vi "DataProcessing.vi"() -> ()   [LabVIEW 2018]
panel:
  out "kat obrotu całkowity":dbl
  out "dystans przebyty x":dbl
  out "kat poł. serwomoechanizmu":dbl
  out "kat pomiaru":dbl
  out "odleglosc pomiaru":dbl
  out "dystans przebyty y":dbl
  out "XY Graph":cluster{dbl[], dbl[]}(graph)
  in  "Port":u16
  in  "Address":string
  in  "stop":bool
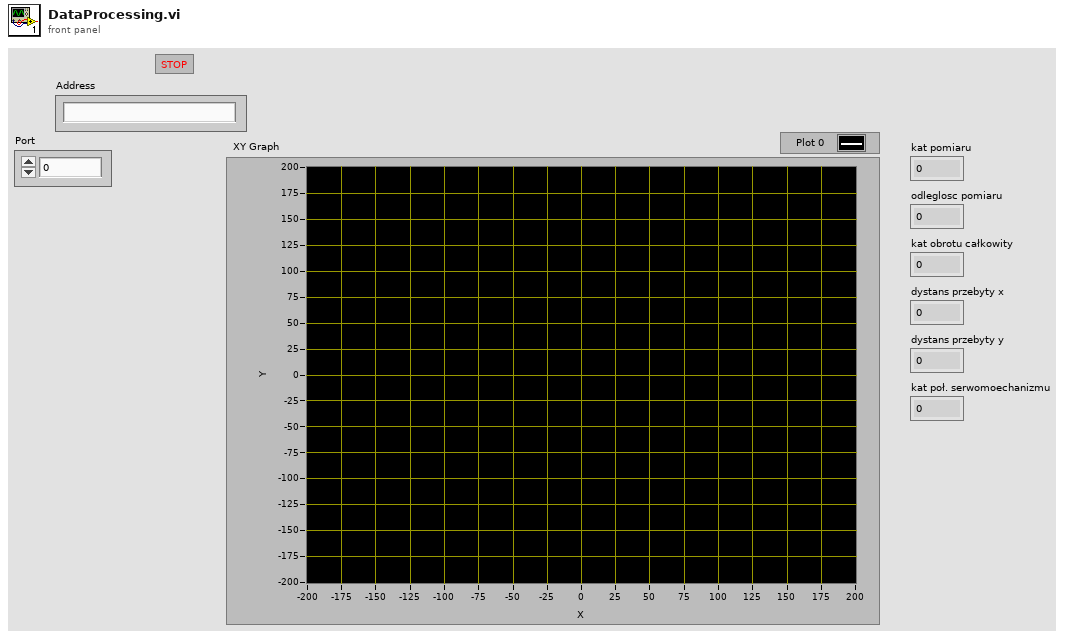
[diagram p1: front panel]
types:
  T1 = enum16{"Standard", "Buffered", "CRLF", "Immediate"}
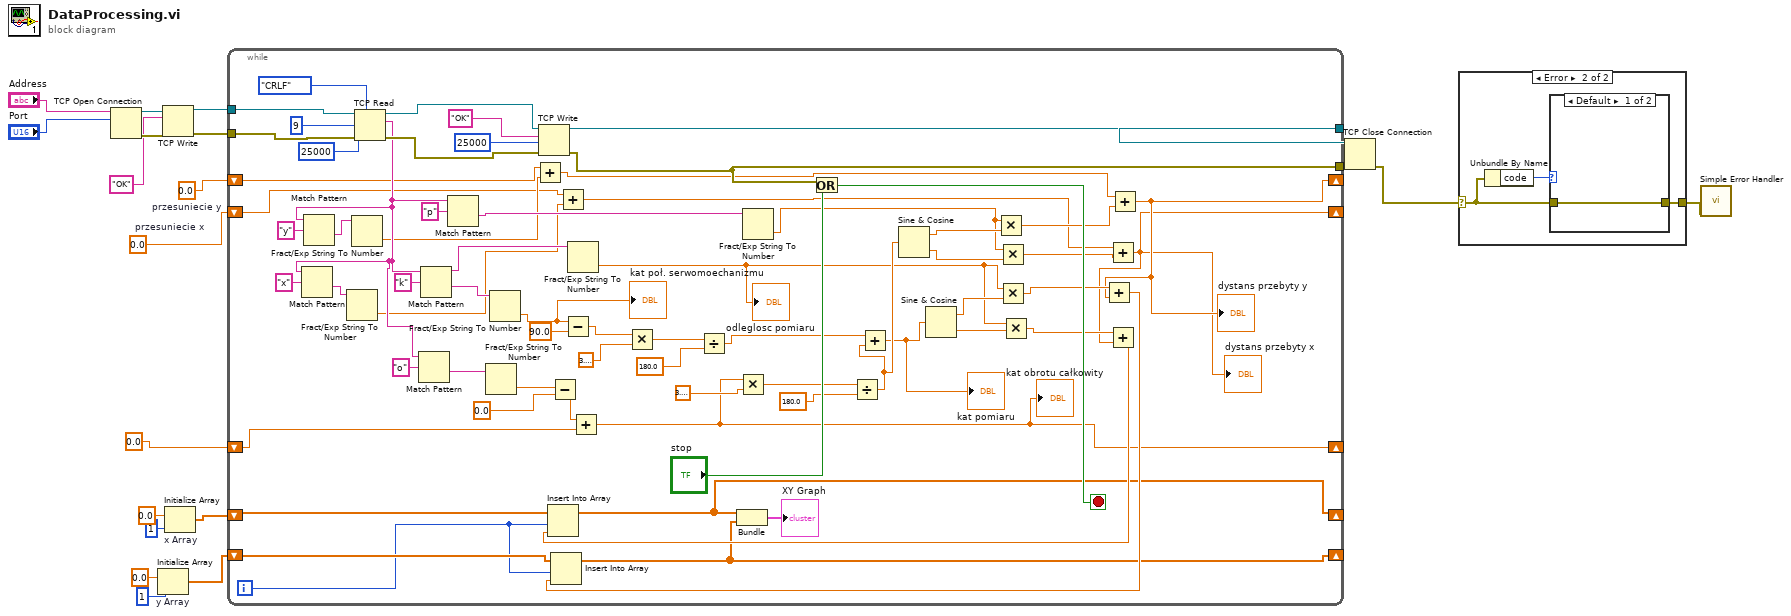
[diagram p0: block diagram]
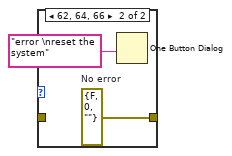
[diagram p3: hidden frame]
diagram:
  w1 = 0.0  # przesuniecie x
  w8 = 0.0  # przesuniecie y
  n1 = TCP Open Connection(address="Address", remote port or service name="Port") -> (connection ID=w16:refnum<k5>, error out=w17:errorcluster)  [unwired: 3 in]
  n2 = Initialize Array "y Array"(0.0 ("element"), 1 ("dimension size")) -> (w3:dbl[])
  n3 = TCP Write(connection ID=w16, data in="OK", error in (no error)=w17) -> (connection ID out=w14:refnum<k5>, error out=w13:errorcluster)  [unwired: 1 in, 1 out]
  n4 = Initialize Array "x Array"(0.0 ("element"), 1 ("dimension size")) -> (w2:dbl[])
  n5 = while {
    tunnel: w14 -> [w82]
    tunnel: w13 -> [w81]
    tunnel: [w78] -> w11
    tunnel: [w77] -> w10
    shift-right: [w32] -> _
    shift-left: 0.0 -> [w66]
    shift-right: [w34] -> _
    shift-left: w8 -> [w26]
    shift-right: [w42] -> _
    shift-left: w2 -> [w48]
    shift-right: [w41] -> _
    shift-left: w3 -> [w47]
    shift-right: [w33] -> _
    shift-left: w1 -> [w23]
    i -> [w46]
    stop <- w79 stop-if-true
    n6 = TCP Read(connection ID=w82, bytes to read=9, error in (no error)=w81, 7:T1."CRLF" ("mode (standard)"), 9:25000 ("timeout ms (25000)")) -> (connection ID out=w76:refnum<k5>, data out=w29:string, error out=w84:errorcluster)
    n7 = Match Pattern(string=w29, regular expression="x") -> (after substring=w27:string)  [unwired: 1 in, 3 out]
    n8 = Match Pattern(string=w29, regular expression="y") -> (after substring=w28:string)  [unwired: 1 in, 3 out]
    n9 = Fract/Exp String To Number(string=w27) -> (number=w22:dbl)  [unwired: 3 in, 1 out]
    n10 = Fract/Exp String To Number(string=w28) -> (number=w25:dbl)  [unwired: 3 in, 1 out]
    n11 = Match Pattern(string=w29, regular expression="o") -> (after substring=w67:string)  [unwired: 1 in, 3 out]
    n12 = Match Pattern(string=w29, regular expression="k") -> (before substring=w58:string, after substring=w74:string)  [unwired: 1 in, 2 out]
    n13 = Match Pattern(string=w29, regular expression="p") -> (after substring=w52:string)  [unwired: 1 in, 3 out]
    n14 = Fract/Exp String To Number(string=w67) -> (number=w64:dbl)  [unwired: 3 in, 1 out]
    n15 = Fract/Exp String To Number(string=w74) -> (number=w38:dbl)  [unwired: 3 in, 1 out]
    "kat poł. serwomoechanizmu" <- w38
    n16 = Add(x=w26, y=w25) -> (x+y=w24:dbl)
    n17 = TCP Write(connection ID=w76, data in="OK", error in (no error)=w84, 9:25000 ("timeout ms (25000)")) -> (connection ID out=w77:refnum<k5>, error out=w78:errorcluster)  [unwired: 1 out]
    n18 = Subtract(x=w64, y=0.0) -> (x-y=w63:dbl)
    n19 = Add(x=w23, y=w22) -> (x+y=w21:dbl)
    n20 = Subtract(x=w38, y=90.0) -> (x-y=w72:dbl)
    n21 = Fract/Exp String To Number(string=w58) -> (number=w40:dbl)  [unwired: 3 in, 1 out]
    "odleglosc pomiaru" <- w40
    n22 = Add(x=w63, y=w66) -> (x+y=w32:dbl)
    "kat obrotu całkowity" <- w32
    n23 = Multiply(x=w72, y=3.141592653589793) -> (x*y=w70:dbl)
    n24 = Divide(x=w70, y=180.0) -> (x/y=w59:dbl)
    n25 = Multiply(x=w32, y=3.141592653589793) -> (x*y=w60:dbl)
    n26 = Fract/Exp String To Number(string=w52) -> (number=w37:dbl)  [unwired: 3 in, 1 out]
    n27 = Or(x=w78, y="stop") -> (x .or. y?=w79:bool)
    n28 = Divide(x=w60, y=180.0) -> (x/y=w51:dbl)
    n29 = Add(x=w59, y=w51) -> (x+y=w39:dbl)
    "kat pomiaru" <- w39
    n30 = Sine & Cosine(0:w51) -> (1:w50:dbl, 2:w49:dbl)
    n31 = Sine & Cosine(0:w39) -> (1:w56:dbl, 2:w57:dbl)
    n32 = Multiply(x=w37, y=w50) -> (x*y=w36:dbl)
    n33 = Multiply(x=w37, y=w49) -> (x*y=w35:dbl)
    n34 = Multiply(x=w40, y=w56) -> (x*y=w55:dbl)
    n35 = Multiply(x=w40, y=w57) -> (x*y=w54:dbl)
    n36 = Add(x=w21, y=w35) -> (x+y=w33:dbl)
    "dystans przebyty x" <- w33
    n37 = Add(x=w54, y=w33) -> (x+y=w44:dbl)
    n38 = Insert Into Array(array=w48, index=w46, new element=w44) -> (w42:dbl[])
    n39 = Add(x=w24, y=w36) -> (x+y=w34:dbl)
    "dystans przebyty y" <- w34
    n40 = Add(x=w55, y=w34) -> (x+y=w45:dbl)
    n41 = Insert Into Array(array=w47, index=w46, new element=w45) -> (w41:dbl[])
    n42 = Bundle(w42, w41) -> (→"XY Graph":cluster{dbl[], dbl[]})  [unwired: 1 in]
  }
  n43 = TCP Close Connection(connection ID=w10, error in (no error)=w11) -> (error out=w12:errorcluster)  [unwired: 1 in, 1 out]
  n44 = case shown="Error" w12 {
    selector: w12 -> [w89 w91]
    tunnel: [w89 w90] -> w20
    frame No Error {
    }
    frame Error {
      n45 = Unbundle By Name(w91) -> ("code"=w92:i32)
      n46 = case shown="Default" w92 {
        tunnel: w91 -> [w93 _]
        tunnel: [w93 w95] -> w90
        frame Default {
        }
        frame 62, 64, 66 {
          w95 = errorcluster {"status"=FALSE, "code"=0, "source"=""}  # No error
          n47 = One Button Dialog(message="error \nreset the system") -> ()  [unwired: 1 in, 1 out]
        }
      }
    }
  }
  n48 = call <vilib>:"Simple Error Handler.vi"("error in (no error)"=w20) -> ()  [unwired: 4 in, 5 out]
